vi "Get all Build Spec Details.vi"(11 "error in (no error)":errorcluster) -> (4 "Build Spec Details":T1[](array[typedef]), 15 "error out":errorcluster)   [LabVIEW 2021, in "Packager Helpers.lvlib"]
uses:
  Packager Helpers.lvlib
  controls/Build Spec Details.ctl
  <vilib>/AppBuilder/AB_API/common/AB_API Build Object Selector.ctl
  <vilib>/AppBuilder/AB_API/Build/NI_AB_API_Build.lvclass
  Dictionary/Dictionary.lvlib
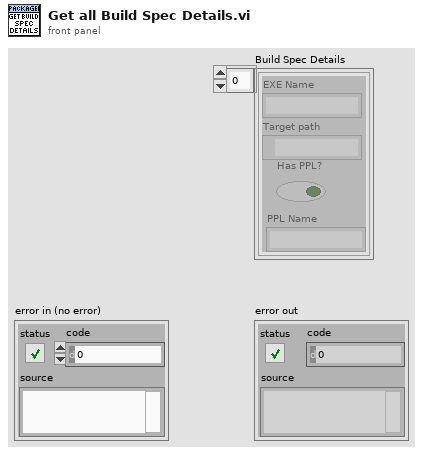
[diagram p1: front panel]
types:
  T1 = typedef "Packager Helpers.lvlib/Build Spec Details.ctl" = cluster{"EXE Name":string, "Target path":path, "Has PPL?":bool, "PPL Name":string}
  T2 = typedef "AB_API Build Object Selector.ctl" = enum16{"Source Distribution", "Deployable Source Distribution", "DLL", "EXE", "Packed Library", "Deployable Packed Library", "RT EXE", ".NET Interop Assembly"}
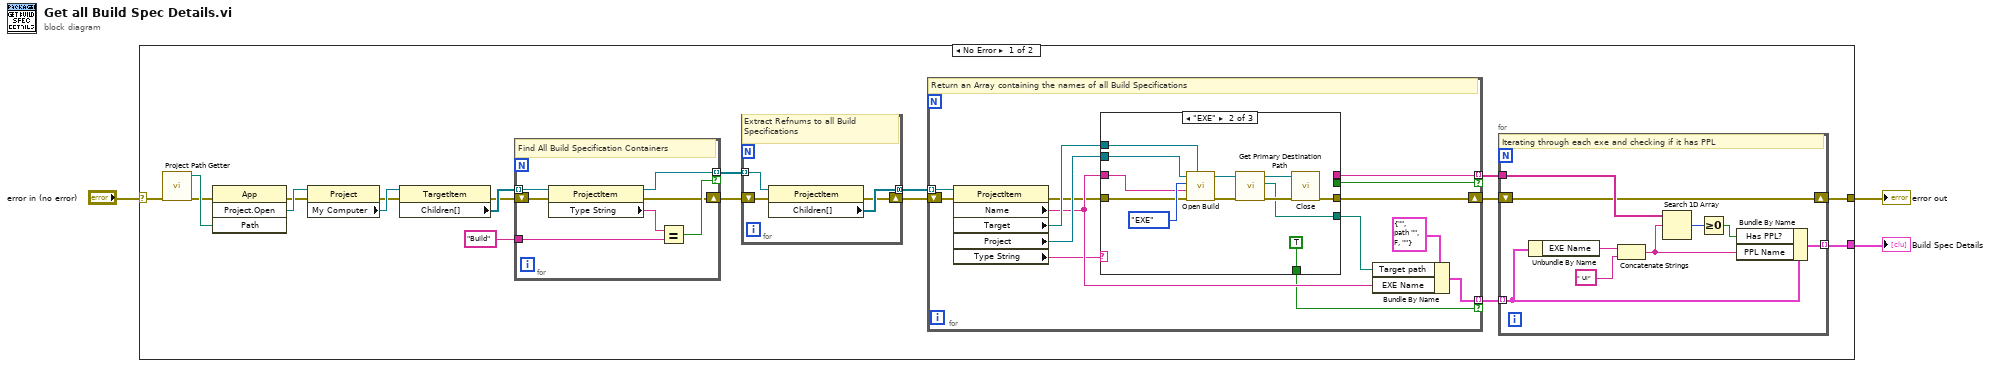
[diagram p0: block diagram]
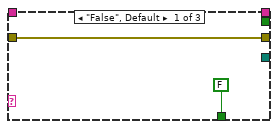
[diagram p2: hidden frame]
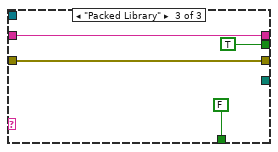
[diagram p3: hidden frame]
diagram:
  n1 = case shown="No Error" "error in (no error)" {
    selector: "error in (no error)" -> [w11 w75]
    tunnel: [w13 w75] -> w3
    tunnel: [w4 _] -> w1
    frame No Error {
      n2 = call "Project Path Getter.vi"("error in (no error)"=w11) -> ("Path"=w12:path, "error out"=w10:errorcluster)  [unwired: 13 in]
      n3 = invoke class="App" method="Project.Open"(error in=w10, "Path"=w12) -> (error out=w9:errorcluster, "Project:Open"=w19:refnum<vi>)  [unwired: 2 in, 2 out]
      n4 = property class="Project"(reference=w19, error in=w9) -> (error out=w8:errorcluster, "My Computer"=w18:refnum<vi>)  [unwired: 1 out]
      n5 = property class="TargetItem"(reference=w18, error in=w8) -> (error out=w7:errorcluster, "Children[]"=w21:refnum<vi>[])  [unwired: 1 out]
      n6 = for {
        tunnel: w21 -> [w65] mode=indexing
        tunnel: [w60] -> w22 mode=indexing if=w64
        shift-right: [w62] -> w17
        shift-left: w7 -> [w63]
        tunnel: "Build" ("y") -> [w59]
        # "Find All Build Specification Containers"
        n7 = property class="ProjectItem"(reference=w65, error in=w63) -> (reference out=w60:refnum<vi>, error out=w62:errorcluster, "Type String"=w61:string)
        n8 = Equal?(x=w61, y=w59) -> (x = y?=w64:bool)
      }
      n9 = for {
        tunnel: w22 -> [w58] mode=indexing
        tunnel: [w57] -> w20 mode=concatenating
        shift-right: [w55] -> w16
        shift-left: w17 -> [w56]
        # "Extract Refnums to all Build Specifications"
        n10 = property class="ProjectItem"(reference=w58, error in=w56) -> (error out=w55:errorcluster, "Children[]"=w57:refnum<vi>[])  [unwired: 1 out]
      }
      n11 = for {
        tunnel: w20 -> [w27] mode=indexing
        shift-right: [w30] -> w15
        shift-left: w16 -> [w33]
        tunnel: [w32] -> w5 mode=indexing if=w26
        tunnel: [w29] -> w14 mode=indexing if=w28
        # "Return an Array containing the names of all Build Specifications"
        n12 = property class="ProjectItem"(reference=w27, error in=w33) -> (error out=w31:errorcluster, "Name"=w34:string, "Target"=w35:refnum<vi>, "Project"=w36:refnum<vi>, "Type String"=w23:string)  [unwired: 1 out]
        n13 = case shown="\"EXE\"" w23 {
          tunnel: [_ w39 _] -> w25
          tunnel: w36 -> [_ w47 _]
          tunnel: w35 -> [_ w46 _]
          tunnel: w34 -> [_ w44 w53]
          tunnel: w31 -> [w38 w42 w54]
          tunnel: [w38 w41 w54] -> w30
          tunnel: [_ _ w53] -> w29
          tunnel: [_ _ TRUE] -> w28
          tunnel: [FALSE TRUE FALSE] -> w26
          frame "False", Default {
          }
          frame "EXE" {
            n14 = call <vilib>:"Open Build.vi"("TargetItem Refnum"=w46, "error in (no error)"=w42, "Build specification name"=w44, "Build object selector"=AB_API_Build_Object_Selector."EXE", "Project Refnum"=w47) -> ("error out"=w43:errorcluster, "NI_AB_API_Build out"=w48:refnum<class "NI_AB_API_Build.lvclass">)  [unwired: 5 in]
            n15 = call-dynamic "Get Primary Destination Path.vi"("error in (no error)"=w43, "NI_AB_API_Build in"=w48) -> ("error out"=w50:errorcluster, "Primary destination path"=w39:path, "NI_AB_API_Build out"=w49:refnum<class "NI_AB_API_Build.lvclass">)  [unwired: 7 in]
            n16 = call-dynamic "Close.vi"("error in (no error)"=w50, "NI_AB_API_Build in"=w49) -> ("error out"=w41:errorcluster)  [unwired: 9 in]
          }
          frame "Packed Library" {
          }
        }
        n17 = Bundle By Name(cluster=T1 {"EXE Name"="", "Target path"=path "", "Has PPL?"=FALSE, "PPL Name"=""}, "Target path"=w25, "EXE Name"=w34) -> (w32:T1)
      }
      n18 = for {
        tunnel: w14 -> [w73]
        shift-right: [w67] -> w13
        shift-left: w15 -> [w67]
        tunnel: w5 -> [w70] mode=indexing
        tunnel: [w66] -> w4 mode=indexing
        # "Iterating through each exe and checking if it has PPL"
        n19 = Unbundle By Name(w70) -> ("EXE Name"=w74:string)
        n20 = Concatenate Strings(w74, " UI" ("string")) -> (w68:string)
        n21 = Search 1D Array(1D array=w73, element=w68) -> (index of element=w72:i32)  [unwired: 1 in]
        n22 = Greater Or Equal To 0?(x=w72) -> (x >= 0?=w71:bool)
        n23 = Bundle By Name(cluster=w70, "Has PPL?"=w71, "PPL Name"=w68) -> (w66:T1)
      }
    }
    frame Error {
    }
  }
  "error out" <- w3
  "Build Spec Details" <- w1
